vi "Retrieve_SetImageProperties.vi"(8 "error in (no error)":errorcluster, 11 "AppImage Properties":T3) -> (0 "error out":errorcluster, 1 "Cancelled?":bool, 2 "Blacklist Out":string[](array[string])=["/var/lib/zerotier-one/identity.public", "/var/lib/zerotier-one/identity.secret"] caption="File and Directory\nBlacklist", 3 "Image Metadata Out":T1 {"component type" items=["standard", "hidden", "system", "unknown", "startup", "image", "essential"]}, 5 "Image Filepath":path)   [LabVIEW 2021]
uses:
  TypeDefs/AppImageProperties.ctl
  TypeDefs/FPGA_Properties_Element.ctl
  <vilib>/nisyscfg/Software 1.2.ctl
  <vilib>/nisyscfg/Component Type.ctl
  <vilib>/Utility/sysdir.llb/System Directory Type.ctl
  <vilib>/nisyscfg/nisyscfg.lvlib
panel:
  in  "Blacklist":string[](array[string])=["/var/lib/zerotier-one/identity.public", "/var/lib/zerotier-one/identity.secret"] caption="File and Directory\nBlacklist"
  in  "Version.Revision":u8
  in  "Version.Minor":u8
  in  "Cancel":bool
  in  "RetireveImg":bool
  in  "Version.Major":u8 caption="Version"
  in  "Description":string
  in  "Title":string
  # "Set Image Properties"
  # "."
  # "."
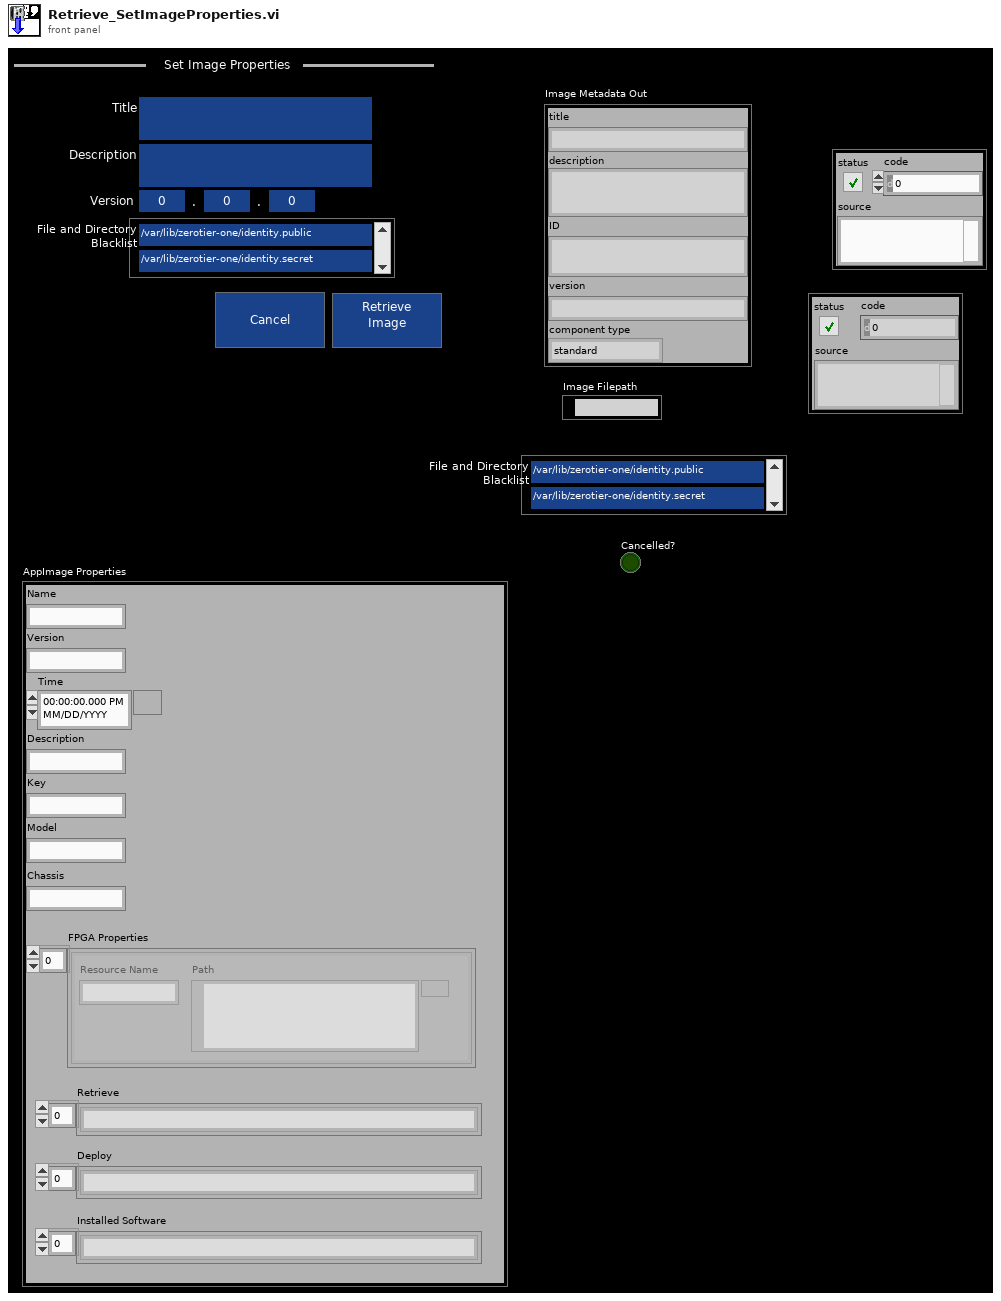
[diagram p1: front panel]
types:
  T1 = typedef "nisyscfg.lvlib/Software 1.2.ctl" = cluster{"title":string, "description":string, "ID":string, "version":string, "component type":T2}
  T2 = typedef "nisyscfg.lvlib/Component Type.ctl" = u32
  T3 = typedef "AppImageProperties.ctl" = cluster{"Name":string, "Version":string, "Time":timestamp, "Description":string, "Key":string, "Chassis":string, "FPGA Properties":T4[], "Model":string, "Retrieve":string[], "Deploy":string[], "Installed Software":string[]}
  T4 = typedef "FPGA_Properties_Element.ctl" = cluster{"Resource Name":string, "Path":path}
  T5 = typedef "System Directory Type.ctl" = i32
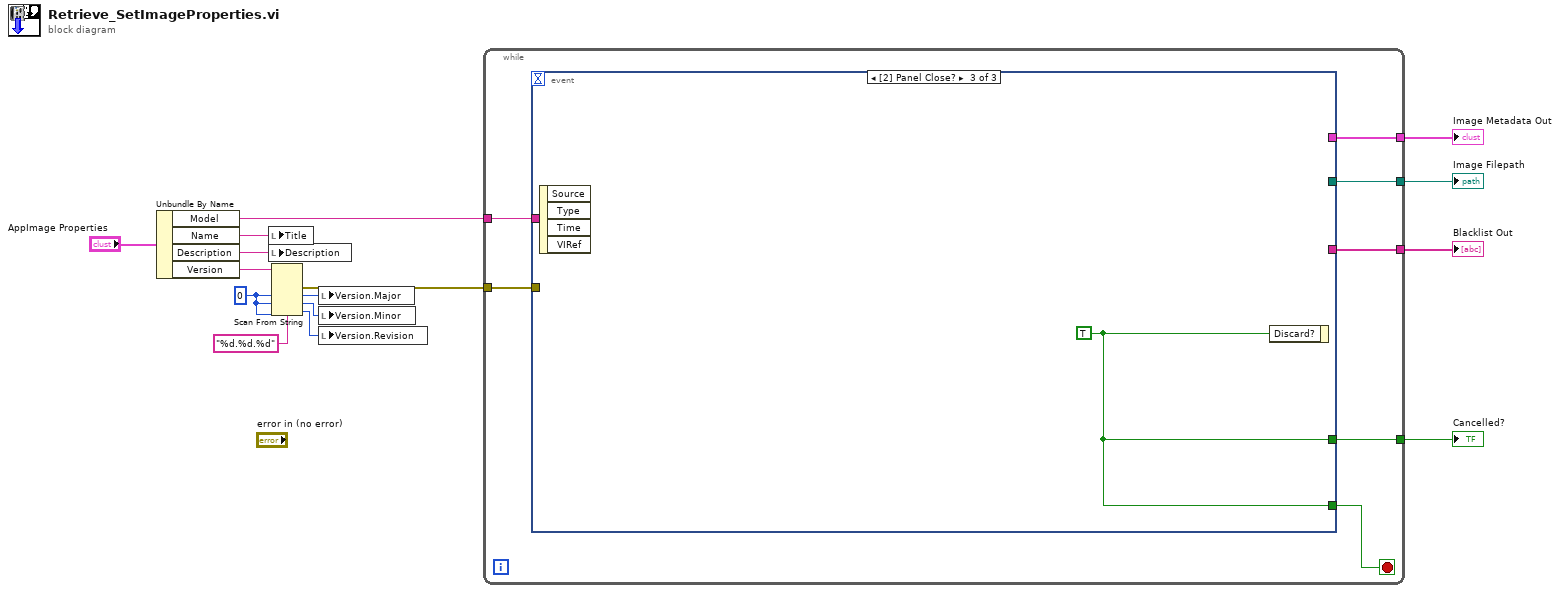
[diagram p0: block diagram]
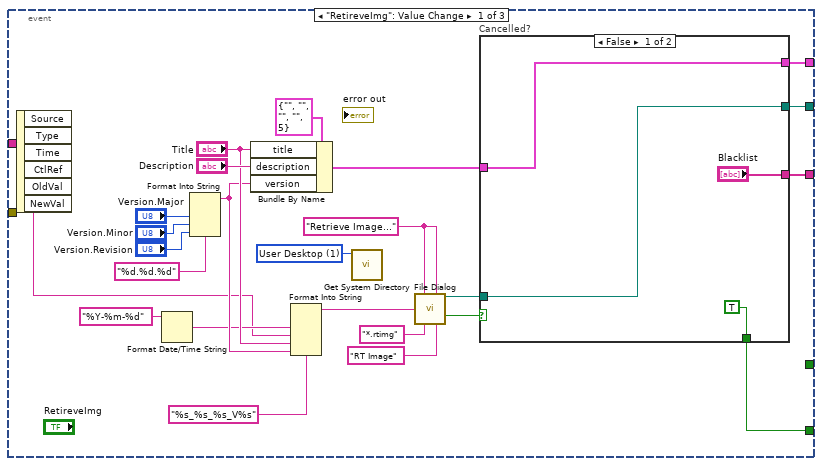
[diagram p2: hidden frame]
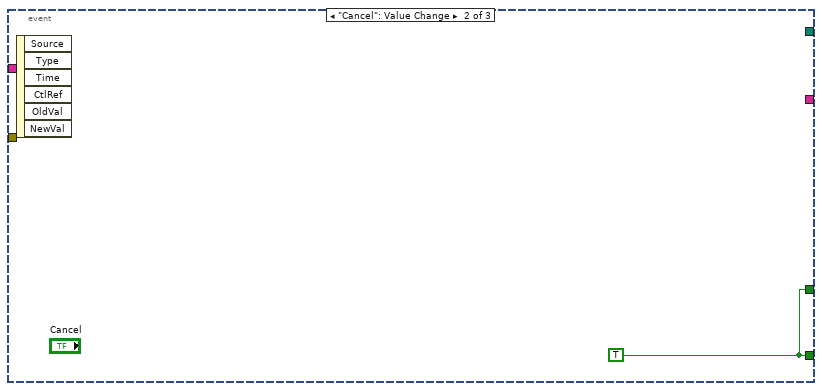
[diagram p4: hidden frame]
diagram:
  w9 = u8 0 ("default value 1")
  n1 = Unbundle By Name("AppImage Properties") -> ("Model"=w1:string, "Name"=w14:string, "Description"=w13:string, "Version"=w11:string)
  n2 = local write "Title"(w14) -> ()
  n3 = local write "Description"(w13) -> ()
  n4 = Scan From String(format string="%d.%d.%d", input string=w11, default 1=w9, default 2=w9, default 3=w9) -> (error out=w6:errorcluster, output 1=w10:u8, output 2=w8:u8, output 3=w7:u8)  [unwired: 2 in, 2 out]
  n5 = local write "Version.Major"(w10) -> ()
  n6 = local write "Version.Minor"(w8) -> ()
  n7 = local write "Version.Revision"(w7) -> ()
  n8 = while {
    tunnel: w6 -> [w22]
    tunnel: [w20] -> w5
    tunnel: [w19] -> w4
    tunnel: [w18] -> w3
    tunnel: [w17] -> w2
    tunnel: w1 -> [w16]
    stop <- w21 stop-if-true
    n9 = event shown="[2] Panel Close?" {
      selector: _ -> [_ _ _]
      dyn-events: _ -> [_ _ _]
      timeout: _ -> [_ _ _]
      tunnel: w22 -> [_ _ _]
      tunnel: [w25 w51 w52] -> w21
      tunnel: [_ w51 w52] -> w20
      tunnel: [w28 _ _] -> w19
      tunnel: [w27 _ _] -> w18
      tunnel: [w26 _ _] -> w17
      tunnel: w16 -> [w23 _ _]
      event "RetireveImg": Value Change {
        w34 = "Retrieve Image..." ("prompt")
        w35 = T5 1 items=["User Home"=0, "User Desktop"=1, "User Documents"=2, "User Application Data"=3, "User Preferences"=4, "User Temporary"=5, "Public Documents"=6, "Public Application Data"=7, "Public Preferences"=8, "Public Cache"=13, "System Core Libraries"=9, "System Installed Libraries"=10, "Application Files"=11, "Boot Volume Root"=12] ("system directory type")
        n10 = event-data() -> ()  [unwired: 1 in, 6 out]
        n11 = Format Date/Time String(time format string (%c)="%Y-%m-%d") -> (date/time string=w24:string)  [unwired: 2 in]
        n12 = Format Into String(format string="%d.%d.%d", "Version.Major", "Version.Minor", "Version.Revision") -> (resulting string=w40:string)  [unwired: 2 in, 1 out]
        n13 = Bundle By Name(cluster=T1 {"title"="", "description"="", "ID"="", "version"="", "component type"=5} ("Image Metadata in"), "title"="Title", "description"="Description", "version"=w40) -> (w31:T1)
        n14 = Format Into String(format string="%s_%s_%s_V%s", w24, w23, "Title", w40) -> (resulting string=w36:string)  [unwired: 2 in, 1 out]
        n15 = call <vilib>:"Get System Directory.vi"("system directory type"=w35) -> ()  [unwired: 10 in, 1 out]
        n16 = call "File Dialog"("prompt"=w34, "button label"=w34, "default name"=w36, "pattern (all files)"="*.rtimg", "pattern label"="RT Image") -> ("selected path"=w30:path, "cancelled"=w29:bool)  [unwired: 7 in, 2 out]
        n17 = case "Cancelled?" shown="False" w29 {
          tunnel: w31 -> [w48 _]
          tunnel: w30 -> [w49 _]
          tunnel: ["Blacklist" _] -> w28
          tunnel: [w49 _] -> w27
          tunnel: [w48 _] -> w26
          tunnel: [TRUE ("Discard?") _] -> w25
          frame False {
          }
          frame True {
          }
        }
      }
      event "Cancel": Value Change {
        w51 = TRUE
        n18 = event-data() -> ()  [unwired: 1 in, 6 out]
      }
      event Panel Close? {
        w52 = TRUE ("Discard?")
        n19 = event-data() -> ()  [unwired: 1 in, 4 out]
        n20 = event-data("Discard?"=w52) -> ()  [unwired: 1 in, 1 out]
      }
    }
  }
  "Cancelled?" <- w5
  "Blacklist Out" <- w4
  "Image Filepath" <- w3
  "Image Metadata Out" <- w2
